vi "Close Connection with CD.vi"(8 "error in":errorcluster, 11 "Comm.Info":T1) -> (0 "error out":errorcluster)   [LabVIEW 2018, in "Instrument Host Automation API.lvlib"]
uses:
  Instrument Host Automation API.lvlib
  <vilib>/NI/STM/NI STM.lvlib
  <vilib>/NI/STM/TCP/Get Connection Reference (TCP).vi
  <vilib>/NI/STM/SubVIs/MetaDataElement.ctl
  <vilib>/NI/STM/TCP/TCP Connection Info.ctl
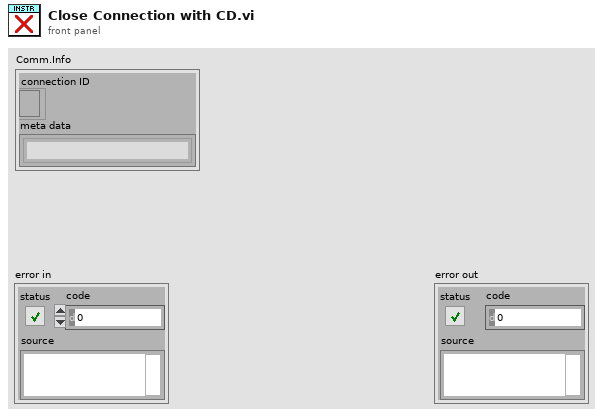
[diagram p1: front panel]
types:
  T1 = typedef "NI STM.lvlib/TCP Connection Info.ctl" = cluster{"connection ID":refnum<k5>, "meta data":T2[]}
  T2 = typedef "NI STM.lvlib/MetaDataElement.ctl" = string
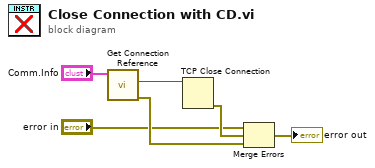
[diagram p0: block diagram]
diagram:
  n1 = call-poly <vilib>:"Get Connection Reference.vi"("connection info in"="Comm.Info") -> ("error out"=w3:errorcluster, "connection ID out"=w5:refnum<k5>)  [unwired: 8 in, 1 out]
  n2 = TCP Close Connection(connection ID=w5) -> (error out=w4:errorcluster)  [unwired: 2 in, 1 out]
  n3 = Merge Errors("error in", w4, w3) -> (→"error out":errorcluster)
